vi "Set Up Dialog - Dissolved Oxygen.vi"() -> ()   [LabVIEW 2012]
panel:
  out "Calibration Instructions":string="1. Connect the sensor to your myDAQ as shown in the diagram above.\n\n2. Once connected, wait 15 mins for the sensor to warm up. \n\n3. Prepare 2 beakers, 1 with diet soda and 1 with tap water. Ensure the volumes are the same.\n\n4. Place the electrode of the DO2N-200E in the beaker with the water. Once the trace settles record the voltage SP2 for 20 % dissolved oxygen. \n\n5. Place the electrode in the beaker with the diet soda. Once the trace settles recrod the voltage for SP1 for 0 % dissolved oxygen."
  # "iWorx - Dissolved Oxygen - Set Up"
  # "Dissolved Oxygen (D02N - 300)"
  # "iWorx"
  # "Sensor"
  # "DO2N - 300"
  # "myDAQ"
  # "Computer"
  # "Adaptor"
  # "Connection Diagram"
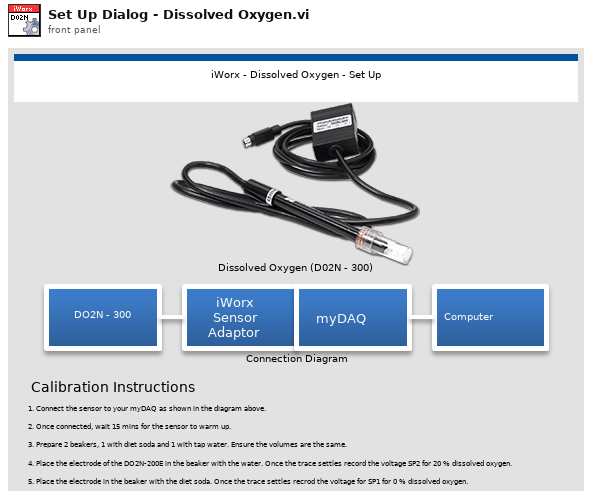
[diagram p1: front panel]
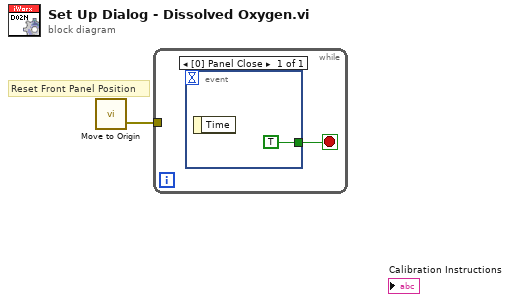
[diagram p0: block diagram]
diagram:
  # "Reset Front Panel Position"
  n1 = call "Move to Origin.vi"() -> ("Error Out"=w1:errorcluster)  [unwired: 3 in]
  n2 = while {
    tunnel: w1 -> [_]
    stop <- w2 stop-if-true
    n3 = event shown="[0] Panel Close" {
      selector: _ -> [_]
      dyn-events: _ -> [_]
      timeout: _ -> [_]
      tunnel: [TRUE] -> w2
      event Panel Close {
        n4 = event-data() -> ()  [unwired: 1 in, 1 out]
      }
    }
  }
